vi "Create listbox IP text - Multi FPGA.vi"(8 "error in (no error)":errorcluster, 10 "ips available":string[](array[string]), 11 "Section Ref in":T1 format="%.0x") -> (0 "error out":errorcluster, 2 "listbox text":string[][](array[string]), 3 "Section Ref out":T1 format="%.0x", 5 "not present item indexes":i32[](array[numeric]))   [LabVIEW 2015, in "Engine Simulation Toolkit System Explorer.lvlib"]
uses:
  Engine Simulation Toolkit System Explorer.lvlib
  <vilib>/NI Veristand/Custom Device API/Custom Device Item Ref.ctl
  Shared/Properties.vi
  <vilib>/NI Veristand/Custom Device API/Get Item Property (String).vi
  Shared/Constants and GUIDs.vi
  <vilib>/NI Veristand/Custom Device API/Get Item Property (String Array).vi
  <vilib>/NI Veristand/Custom Device API/Custom Device API.lvlib
  Shared/Engine Simulation Toolkit Shared.lvlib
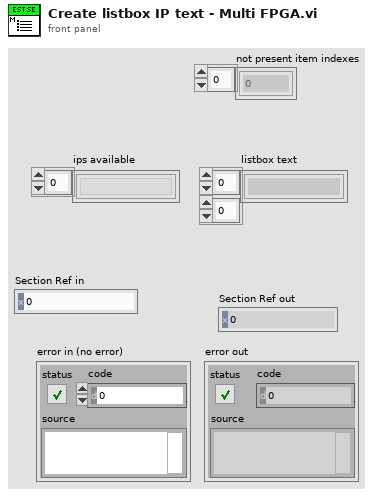
[diagram p1: front panel]
types:
  T1 = typedef "Custom Device API.lvlib/Custom Device Item Ref.ctl" = u64
  T2 = typedef "Custom Device API.lvlib/Custom Device Item Info.ctl" = cluster{"Name":string, "Is Channel":bool, "GUID":string, "Is Waveform":bool}
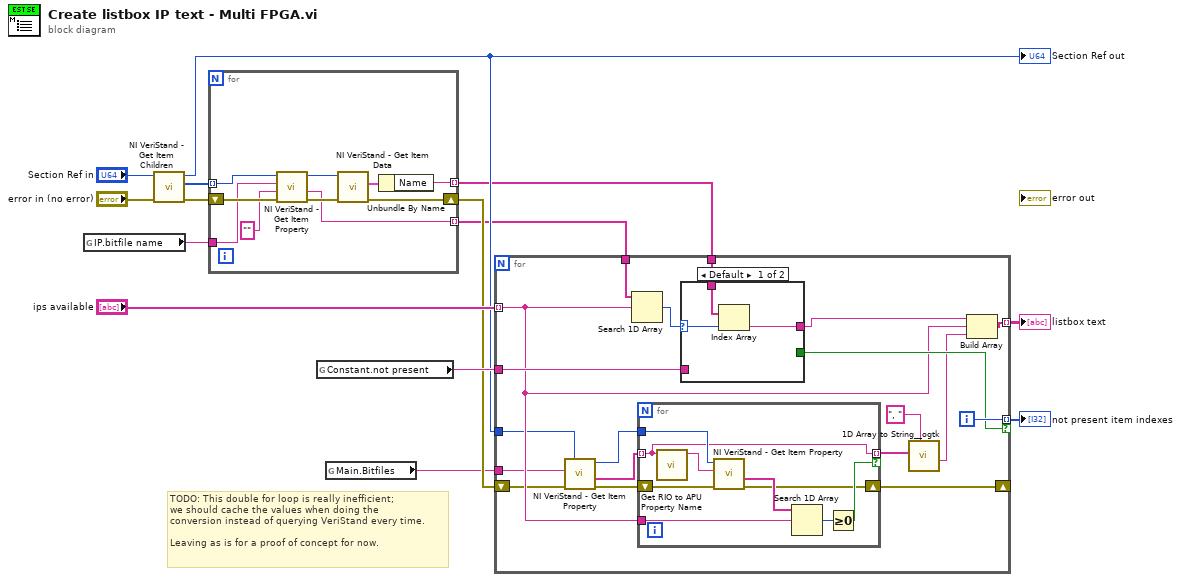
[diagram p0: block diagram]
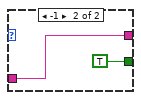
[diagram p2: hidden frame]
diagram:
  # "TODO: This double for loop is really inefficient;\nwe should cache the values when doing the\nconversion instead of querying VeriStand every time.\n\nLeaving as is for a proof of concept for now."
  n1 = global read "Properties.vi" "IP.bitfile name"() -> (w10:string)
  n2 = call <vilib>:"NI VeriStand - Get Item Children.vi"("error in (no error)"="error in (no error)", "Item Ref in"="Section Ref in") -> ("error out"=w12:errorcluster, "Child Refs"=w11:T1[], "Item Ref out"=w4:T1)  [unwired: 6 in, 1 out]
  "Section Ref out" <- w4
  n3 = for {
    shift-right: [w19] -> w5
    shift-left: w12 -> [w24]
    tunnel: w11 -> [w22] mode=indexing
    tunnel: w10 -> [w21]
    tunnel: [w16] -> w2 mode=indexing
    tunnel: [w15] -> w1 mode=indexing
    n4 = call-poly <vilib>:"NI VeriStand - Get Item Property.vi"("error in (no error)"=w24, "Default Value"="", "Property Name"=w21, "Item Ref in"=w22) -> ("error out"=w23:errorcluster, "Value"=w16:string, "Item Ref out"=w18:T1)  [unwired: 4 in, 1 out]
    n5 = call <vilib>:"NI VeriStand - Get Item Data.vi"("error in (no error)"=w23, "Item Ref in"=w18) -> ("error out"=w19:errorcluster, "Item Info"=w17:T2)  [unwired: 6 in, 2 out]
    n6 = Unbundle By Name(w17) -> ("Name"=w15:string)
  }
  n7 = global read "Constants and GUIDs.vi" "Constant.not present"() -> (w7:string)
  n8 = global read "Properties.vi" "Main.Bitfiles"() -> (w3:string)
  n9 = for {
    tunnel: "ips available" -> [w35] mode=indexing
    tunnel: w2 -> [w36]
    tunnel: w1 -> [w42]
    tunnel: [w40] -> w8 mode=indexing
    tunnel: w7 -> [w39]
    tunnel: [w38] -> w6 mode=indexing if=w37
    shift-right: [w31] -> _
    shift-left: w5 -> [w30]
    tunnel: w4 -> [w28]
    tunnel: w3 -> [w25]
    i -> [w38]
    n10 = call-poly <vilib>:"NI VeriStand - Get Item Property.vi"("error in (no error)"=w30, "Property Name"=w25, "Item Ref in"=w28) -> ("error out"=w29:errorcluster, "Value"=w26:string[], "Item Ref out"=w27:T1)  [unwired: 5 in, 1 out]
    n11 = Search 1D Array(1D array=w36, element=w35) -> (index of element=w43:i32)  [unwired: 1 in]
    n12 = for {
      tunnel: w35 -> [w50]
      tunnel: [w44] -> w33 mode=indexing if=w49
      shift-right: [w47] -> w31
      shift-left: w29 -> [w48]
      tunnel: w27 -> [w46]
      tunnel: w26 -> [w44] mode=indexing
      n13 = call "Get RIO to APU Property Name.vi"("rio name"=w44) -> ("property name"=w45:string)  [unwired: 10 in]
      n14 = call-poly <vilib>:"NI VeriStand - Get Item Property.vi"("error in (no error)"=w48, "Property Name"=w45, "Item Ref in"=w46) -> ("error out"=w47:errorcluster, "Value"=w52:string[])  [unwired: 5 in, 2 out]
      n15 = Search 1D Array(1D array=w52, element=w50) -> (index of element=w51:i32)  [unwired: 1 in]
      n16 = Greater Or Equal To 0?(x=w51) -> (x >= 0?=w49:bool)
    }
    n17 = case shown="Default" w43 {
      selector: w43 -> [w54 _]
      tunnel: [w53 w57] -> w41
      tunnel: w42 -> [w55 _]
      tunnel: w39 -> [_ w57]
      tunnel: [_ TRUE] -> w37
      frame Default {
        n18 = Index Array(array=w55, index=w54) -> (element=w53:string)
      }
      frame -1 {
      }
    }
    n19 = call <userlib>:"1D Array to String__ogtk.vi"("delimiter (Tab)"=", ", "Array of Strings"=w33) -> ("delimited string"=w32:string)  [unwired: 9 in]
    n20 = Build Array(w41, w35, w32) -> (w40:string[])
  }
  "listbox text" <- w8
  "not present item indexes" <- w6
